vi "THz Time(SR830_VC_PSD)_TA_170401.vi"(4 "Lockin Address":string="12") -> ()   [LabVIEW 2010]
panel:
  in  "CONEX-PSD9 Instrument Key 2":string="CONEX-PSD (A6ULD73M)"
  in  "Exit Program":bool
  out "Y position":dbl=-5.0 format="%#.3p"
  out "X position":dbl=-5.0 format="%#.3p"
  out "Power meter":dbl format="%#.3p"
  in  "Launch server?":bool
  in  "Authorize?":bool=TRUE
  out "error out":errorcluster
  out "Position 2":dbl[](array[numeric])=[2.395] format="%.6f"
  in  "error in":errorcluster
  out "Running":bool caption="Mercury_GCS_Configuration_Setup.vi is running"
  out "Conn. Axis":string[](array[string])=["1"]
  out "Identification":string="(c)2013 Physik Instrumente(PI) Karlsruhe, C-863.11,0,1.3.0.7"
  in  "SaveFile name":string="t"
  in  "Interdelay (ms)":dbl=10.0
  in  "pre delay (ms)":dbl=100.0
  out "Lock-in Y-Channel":dbl=-7.0941e-11 format="%#.3p"
  out "Lock-in X-Channel":dbl=5.62071e-10 format="%#.3p"
  out "THz Time-domain Signal Wave":cluster{"x-axis":sgl[], "y-axis":dbl[]}(graph)={"x-axis"=[3.4, 3.395, 3.39, 3.385, 3.38, 3.375, 3.3700001, 3.365, 3.3600001, 3.355, 3.3500001, 3.345, 3.3400002, 3.335, 3.3300002, 3.325, 3.3200002, 3.315, 3.3100002, 3.305, 3.3000002, 3.295, 3.2900002, 3.285, 3.2800002, 3.275, 3.27, 3.265, 3.26, 3.255, 3.25, 3.2450001, 3.24, 3.2350001, 3.23, 3.2250001, 3.22, 3.2150002, 3.21, 3.2050002, 3.2, 3.1950002, 3.19, 3.1850002, 3.18, 3.1750002, 3.17, 3.1650002, 3.16, 3.1550002, 3.15, 3.1450002, 3.14, 3.135, 3.13, 3.125, 3.1200001, 3.115, 3.1100001, 3.105, 3.1000001, 3.095, 3.0900002, 3.085, 3.0800002, 3.075, 3.0700002, 3.065, 3.0600002, 3.055, 3.0500002, 3.045, 3.0400002, 3.035, 3.0300002, 3.025, 3.0200002, 3.015, 3.01, 3.005, 3.0, 2.9950001, 2.99, 2.9850001, 2.98, 2.9750001, 2.97, 2.9650002, 2.96, 2.9550002, 2.95, 2.9450002, 2.94, 2.9350002, 2.93, 2.9250002, 2.92, 2.9150002, 2.91, 2.9050002, 2.9, 2.8950002, 2.89, 2.885, 2.88, 2.875, 2.8700001, 2.865, 2.8600001, 2.855, 2.8500001, 2.845, 2.8400002, 2.835, 2.8300002, 2.825, 2.8200002, 2.815, 2.8100002, 2.805, 2.8000002, 2.795, 2.7900002, 2.785, 2.7800002, 2.775, 2.7700002, 2.765, 2.7600002, 2.755, 2.75, 2.7450001, 2.74, 2.7350001, 2.73, 2.7250001, 2.72, 2.7150002, 2.71, 2.7050002, 2.7, 2.6950002, 2.69, 2.6850002, 2.68, 2.6750002, 2.67, 2.6650002, 2.66, 2.6550002, 2.65, 2.6450002, 2.64, 2.6350002, 2.63, 2.625, 2.6200001, 2.615, 2.6100001, 2.605, 2.6000001, 2.595, 2.5900002, 2.585, 2.5800002, 2.575, 2.5700002, 2.565, 2.5600002, 2.555, 2.5500002, 2.545, 2.5400002, 2.535, 2.5300002, 2.525, 2.5200002, 2.515, 2.5100002, 2.505, 2.5, 2.4950001, 2.49, 2.4850001, 2.48, 2.4750001, 2.47, 2.4650002, 2.46, 2.4550002, 2.45, 2.4450002, 2.44, 2.4350002, 2.43, 2.4250002, 2.42, 2.4150002, 2.41, 2.4050002, 2.4, 2.3950002], "y-axis"=array[202 elements]}
  in  "Autosave Directory for Long-term Average Scan":path=path "D:/Soon/140901_delay_test/2_VC_delay_ESP_-2.35/1_VC_delay"
  in  "OK Button":bool
  out "Data Type":string="outp ? 1"
  in  "Enum":enum16{"X", "Y", "Abs"}(ring)
  in  "SCAN":bool
  in  "Short term \nAverage#":i8=2
  in  "Step":sgl=0.005 min=0 max=10000 format="%.3f"
  in  "End Postion":sgl=2.4 min=-400 max=400 format="%#.3f"
  in  "Start Position":sgl=3.4 min=-400 max=400 format="%#.3f"
  # "This Program Run First (1) and then Run the Approach Program (2)"
  # "THz Experiment"
  # "``"
  # "Input Data"
  # "Auto-offset"
  # "Point Avg"
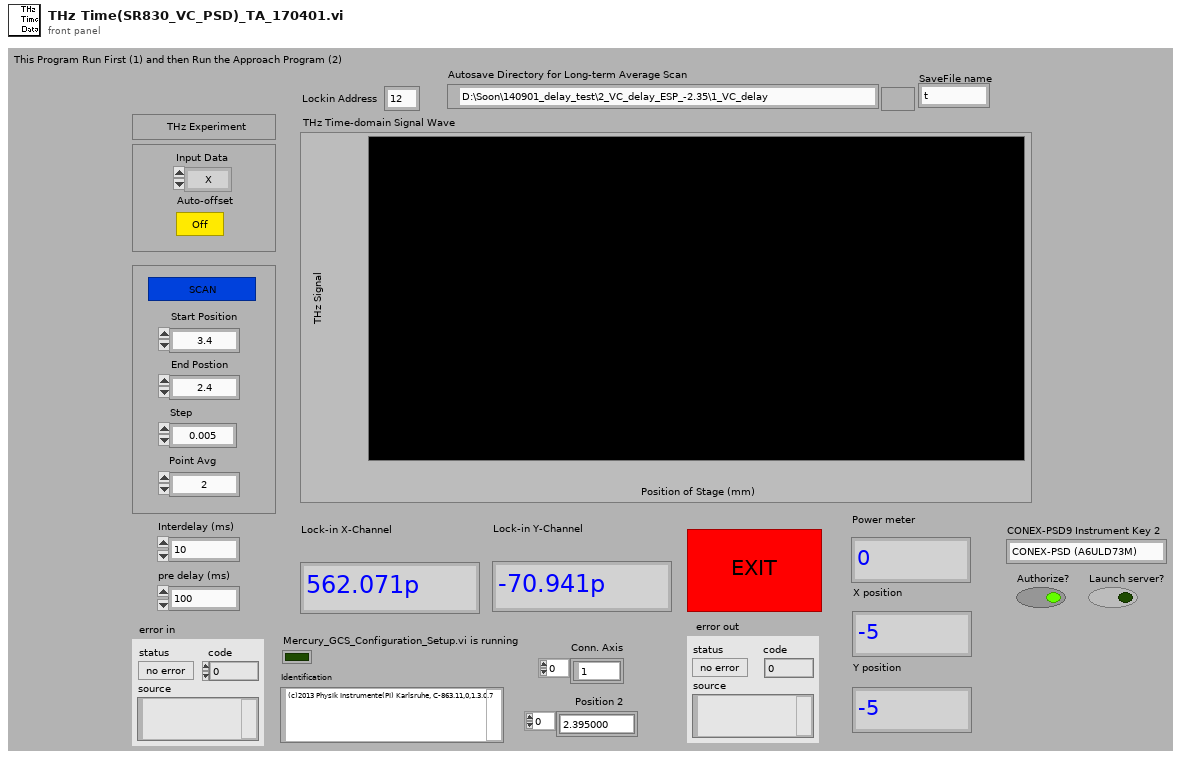
[diagram p1: front panel]
types:
  T1 = cluster{"ConexPSD Reference":refnum<k24>, "error out":errorcluster, "Component ID":i32}
  T2 = cluster{"System no.":i32, "error out":errorcluster}
  T3 = cluster{"Step Number":i32, "Step":sgl, "Start Position":sgl, "Time-out":i32, "Lockin Address":string, "Short term \nAverage#":i8, "System no.":i32, "error out":errorcluster, "Value":string, "pre delay (ms)":dbl, "Interdelay (ms)":dbl, "Autosave Directory for Long-term Average Scan":path, cluster{"ConexPSD Reference":refnum<k24>, "error out":errorcluster, "Component ID":i32}}
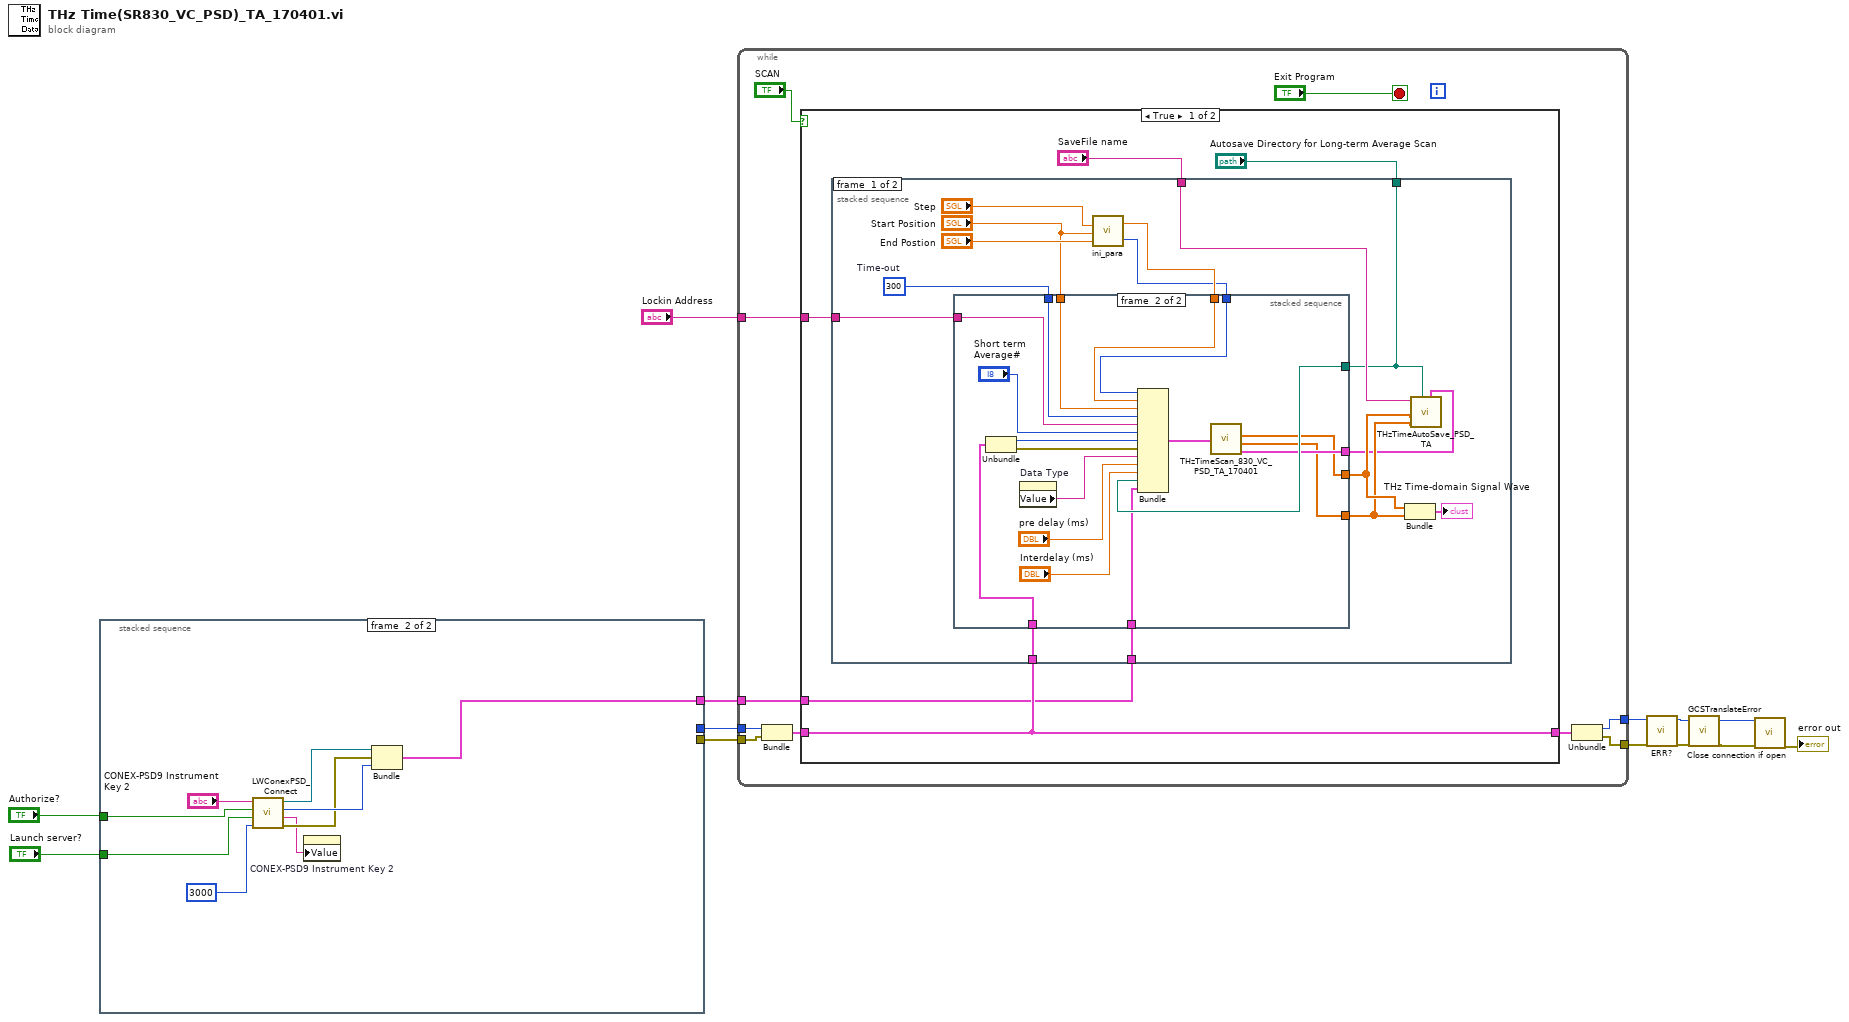
[diagram p0: block diagram]
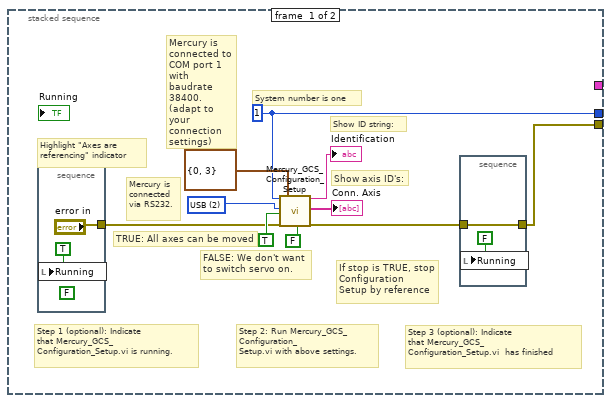
[diagram p2: hidden frame]
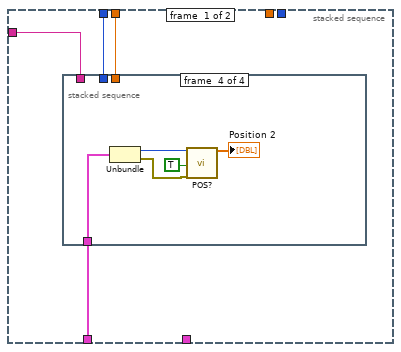
[diagram p3: hidden frame]
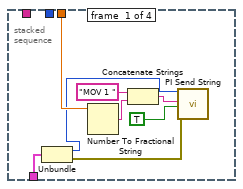
[diagram p4: hidden frame]
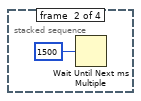
[diagram p5: hidden frame]
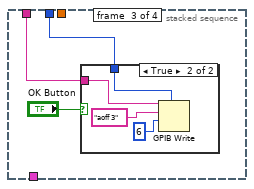
[diagram p6: hidden frame]
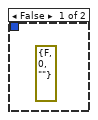
[diagram p7: hidden frame]
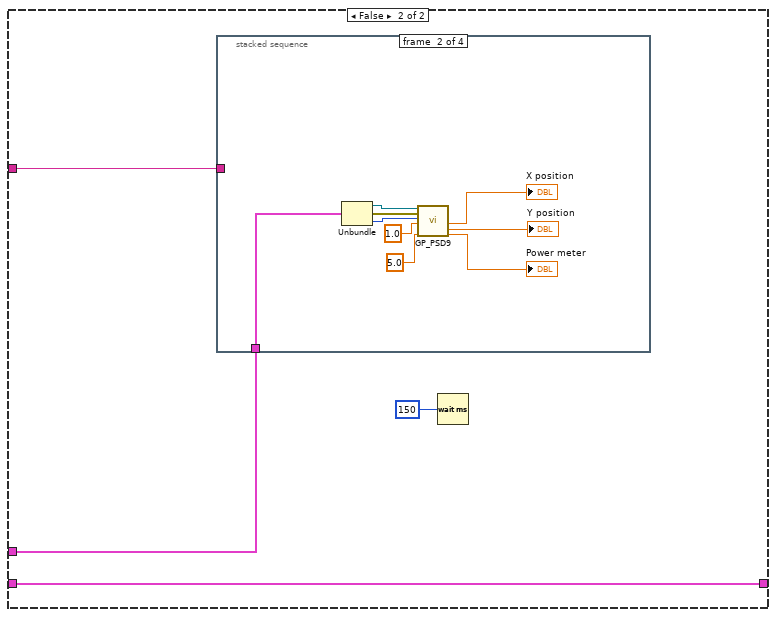
[diagram p9: hidden frame]
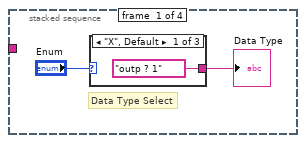
[diagram p10: hidden frame]
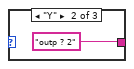
[diagram p11: hidden frame]
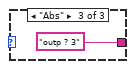
[diagram p12: hidden frame]
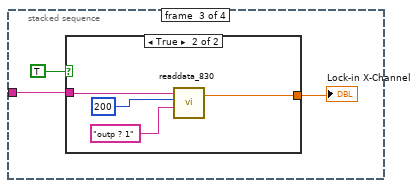
[diagram p13: hidden frame]
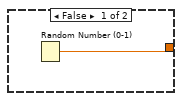
[diagram p14: hidden frame]
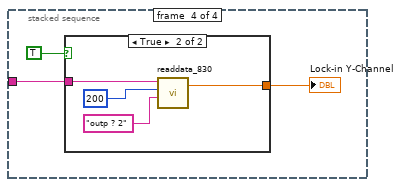
[diagram p15: hidden frame]
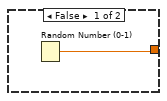
[diagram p16: hidden frame]
diagram:
  n1 = stacked-sequence {
    tunnel: [w13 _] -> w10
    tunnel: [w12 _] -> w9
    tunnel: "Authorize?" -> [_ w28]
    tunnel: "Launch server?" -> [_ w27]
    tunnel: [_ w26] -> w1
    frame #0 {
      w14 = u16 2 items=["RS232", "RS232 DaisyChain", "USB", "USB_DaisyChain"] ("Interface")
      w13 = 1 ("System no.")
      # "Mercury is\nconnected\nvia RS232."
      # "If stop is TRUE, stop \nConfiguration\nSetup by reference"
      # "Mercury is\nconnected to\nCOM port 1\nwith baudrate\n38400.\n(adapt to your\nconnection\nsettings)"
      # "Step 3 (optional): Indicate\nthat Mercury_GCS_\nConfiguration_Setup.vi  has finished"
      # "Step 2: Run Mercury_GCS_\nConfiguration_\nSetup.vi with above settings."
      # "Step 1 (optional): Indicate\nthat Mercury_GCS_\nConfiguration_Setup.vi is running."
      # "Highlight \"Axes are\nreferencing\" indicator"
      # "Show axis ID's:"
      # "Show ID string:"
      # "FALSE: We don't want\nto switch servo on."
      # "TRUE: All axes can be moved"
      # "System number is one"
      n2 = stacked-sequence {
        tunnel: ["error in"] -> w17
        frame #0 {
          (unwired) FALSE ("stop")
          n3 = local write "Running"(TRUE ("Running")) -> ()
        }
      }
      n4 = call "Mercury_GCS_Configuration_Setup.vi"("System no."=w13, "Interface"=w14, "All axes?"=TRUE, "error in"=w17, "RS232 settings"=cluster{"RS232 Portnumber":i32, "Baudrate":u16} {"RS232 Portnumber"=0, "Baudrate"=3}, "Switch servo on?"=FALSE ("Use dialog to define\nconnected stages?")) -> ("Identification"=→"Identification":string, "Conn. \nAxes"=→"Conn. Axis":string[], "error out"=w18:errorcluster)  [unwired: 7 in, 4 out]
      n5 = stacked-sequence {
        tunnel: w18 -> [w25]
        tunnel: [w25] -> w12
        frame #0 {
          n6 = local write "Running"(FALSE ("Running")) -> ()
        }
      }
    }
    frame #1 {
      n7 = call "LWConexPSD_Connect.vi"("DiscoverTimeout (10000 msec)"=3000, "Launch server? (True)"=w27, "Authorize? (True)"=w28, "Instrument Key"="CONEX-PSD9 Instrument Key 2") -> ("error out"=w32:errorcluster, "Instrument Key out"=w30:string, "Component ID"=w33:i32, "ConexPSD Reference"=w31:refnum<k24>)
      n8 = property on="CONEX-PSD9 Instrument Key 2" class="Str"("Value"=w30) -> ()  [unwired: 2 in, 2 out]
      n9 = Bundle("ConexPSD Reference"=w31, "error out"=w32, "Component ID"=w33) -> (w26:T1)  [unwired: 1 in]
    }
  }
  n10 = while {
    tunnel: "Lockin Address" -> [w43]
    tunnel: w10 -> [w42]
    tunnel: w9 -> [w41]
    tunnel: [w38] -> w5
    tunnel: [w37] -> w4
    tunnel: w1 -> [w35]
    stop <- "Exit Program" stop-if-true
    n11 = Bundle("System no."=w42, "error out"=w41) -> (w40:T2)  [unwired: 1 in]
    n12 = case shown="True" "SCAN" {
      tunnel: w43 -> [w49 w110]
      tunnel: w40 -> [w48 w109]
      tunnel: [w48 w109] -> w39
      tunnel: w35 -> [w45 w108]
      frame True {
        n13 = stacked-sequence {
          tunnel: w49 -> [w60 _]
          tunnel: "SaveFile name" -> [w52 _]
          tunnel: w48 -> [w59 _]
          tunnel: "Autosave Directory for Long-term Average Scan" -> [w51 _]
          tunnel: w45 -> [w55 _]
          frame #0 {
            w64 = 300  # Time-out
            n14 = call "ini_para.vi"("End Position"="End Postion", "Start Position"="Start Position", "Step"="Step") -> ("Step Number"=w56:i32, "Step"=w57:sgl)
            n15 = stacked-sequence {
              tunnel: w64 -> [w68 w106]
              tunnel: "Start Position" -> [w67 w98]
              tunnel: w57 -> [_ w99]
              tunnel: w56 -> [_ w107]
              tunnel: [_ w91] -> w54
              tunnel: [_ w90] -> w53
              tunnel: w51 -> [_ w101]
              tunnel: w60 -> [w66 w100]
              tunnel: w59 -> [w65 w97]
              tunnel: w55 -> [_ w94]
              tunnel: [_ w93] -> w50
              frame #0 {
                n16 = stacked-sequence {
                  tunnel: w68 -> [_ _ w79 _]
                  tunnel: w67 -> [w72 _ _ _]
                  tunnel: w66 -> [_ _ w78 _]
                  tunnel: w65 -> [w71 _ _ w87]
                  frame #0 {
                    n17 = Unbundle(w71) -> ("System no."=w69:i32, "error out"=w70:errorcluster)
                    n18 = Number To Fractional String(number=w72) -> (F-format string=w73:string)  [unwired: 3 in]
                    n19 = Concatenate Strings("MOV 1 ", w73) -> (w76:string)
                    n20 = call "PI Send String.vi"("System no."=w69, "String to send"=w76, "Attach termination char.?"=TRUE ("Attach Linefeed?"), "error in"=w70) -> ()  [unwired: 15 in, 1 out]
                  }
                  frame #1 {
                    n21 = Wait Until Next ms Multiple(millisecond multiple=1500) -> ()  [unwired: 1 out]
                  }
                  frame #2 {
                    n22 = case shown="True" "OK Button" {
                      tunnel: w79 -> [_ w83]
                      tunnel: w78 -> [_ w81]
                      frame False {
                        (unwired) errorcluster {"status"=FALSE, "code"=0, "source"=""} ("error in")
                      }
                      frame True {
                        n23 = GPIB Write(0:w81, 1:"aoff 3" ("data"), 2:i16 6 ("mode (0)"), 4:w83) -> ()  [unwired: 1 in, 2 out]
                      }
                    }
                  }
                  frame #3 {
                    n24 = Unbundle(w87) -> ("System no."=w86:i32, "error out"=w85:errorcluster)
                    n25 = call "POS?.vi"("System no."=w86, "All axes?"=TRUE, "error in"=w85) -> ("Position"=→"Position 2":dbl[])  [unwired: 15 in, 1 out]
                  }
                }
              }
              frame #1 {
                n26 = Unbundle(w97) -> ("System no."=w96:i32, "error out"=w95:errorcluster)
                n27 = property on="Data Type" class="Str"() -> ("Value"=w104:string)  [unwired: 2 in, 2 out]
                n28 = Bundle("Step Number"=w107, "Step"=w99, "Start Position"=w98, "Time-out"=w106, "Lockin Address"=w100, "Short term \nAverage#"="Short term \nAverage#", "System no."=w96, "error out"=w95, "Value"=w104, "pre delay (ms)"="pre delay (ms)", "Interdelay (ms)"="Interdelay (ms)", "Autosave Directory for Long-term Average Scan"=w101, w94) -> (w92:T3)  [unwired: 1 in]
                n29 = call "THzTimeScan_830_VC_PSD_TA_170401.vi"("input"=w92) -> ("x-axis"=w91:sgl[], "y-axis"=w90:dbl[], "ext. out"=w93:cluster{dbl[], dbl[], dbl[], dbl[], string[]})  [unwired: 1 out]
              }
            }
            n30 = Bundle("x-axis"=w54, "y-axis"=w53) -> (→"THz Time-domain Signal Wave":cluster{"x-axis":sgl[], "y-axis":dbl[]})  [unwired: 1 in]
            n31 = call "THzTimeAutoSave_PSD_TA.vi"("ext. out"=w50, "Autosave Directory for Long-term Average Scan"=w51, "y-axis"=w53, "x-axis"=w54, "SaveFile name"=w52) -> ()  [unwired: 5 in]
          }
          frame #1 {
          }
        }
      }
      frame False {
        n32 = stacked-sequence {
          tunnel: w110 -> [_ _ w126 w135]
          tunnel: w108 -> [_ w120 _ _]
          frame #0 {
            # "Data Type Select"
            n33 = case shown="\"X\", Default" "Enum" {
              tunnel: ["outp ? 1" "outp ? 2" "outp ? 3"] -> w113
              frame "X", Default {
              }
              frame "Y" {
              }
              frame "Abs" {
              }
            }
            "Data Type" <- w113
          }
          frame #1 {
            n34 = Unbundle(w120) -> ("ConexPSD Reference"=w125:refnum<k24>, "error out"=w124:errorcluster, "Component ID"=w123:i32)
            n35 = call "GP_PSD9.vi"("ConexPSD Reference"=w125, "error out"=w124, "Component ID"=w123, "Adress"=1.0 ("shot average"), "shot average"=5.0) -> ("PositionX"=→"X position":dbl, "PositionY"=→"Y position":dbl, "LaserPower"=→"Power meter":dbl)  [unwired: 8 in, 4 out]
          }
          frame #2 {
            n36 = case shown="True" TRUE {
              tunnel: [w129 w131] -> w128
              tunnel: w126 -> [_ w130]
              frame False {
                n37 = Random Number (0-1)() -> (number: 0 to 1=w129:dbl)
              }
              frame True {
                n38 = call "readdata_830.vi"("Command"="outp ? 1", "timeout"=200, "Lockin Address"=w130) -> ("Data"=w131:dbl)  [unwired: 1 in, 1 out]
              }
            }
            "Lock-in X-Channel" <- w128
          }
          frame #3 {
            n39 = case shown="True" TRUE {
              tunnel: w135 -> [_ w139]
              tunnel: [w137 w138] -> w134
              frame False {
                n40 = Random Number (0-1)() -> (number: 0 to 1=w137:dbl)
              }
              frame True {
                n41 = call "readdata_830.vi"("Command"="outp ? 2", "timeout"=200, "Lockin Address"=w139) -> ("Data"=w138:dbl)  [unwired: 1 in, 1 out]
              }
            }
            "Lock-in Y-Channel" <- w134
          }
        }
        n42 = Wait (ms)(milliseconds to wait=u32 150) -> ()  [unwired: 1 out]
      }
    }
    n43 = Unbundle(w39) -> ("System no."=w38:i32, "error out"=w37:errorcluster)
  }
  n44 = call "ERR?.vi"("error in"=w4) -> ("error out"=w7:errorcluster)  [unwired: 17 in, 1 out]
  n45 = call "GCSTranslateError.vi"("error in"=w7) -> ("error out"=w6:errorcluster)  [unwired: 16 in, 2 out]
  n46 = call "Close connection if open.vi"("System no."=w5, "error in"=w6) -> ("error out"=→"error out":errorcluster)  [unwired: 16 in, 1 out]
